vi "NI VeriStand - Timing Engine Globals.vi"() -> ()   [LabVIEW 2010, in "NI_VS FPGA Clock Support.lvlib"]
uses:
  <userlib>/_NI VeriStand FPGA Support/NI VeriStand FPGA Clock Support/NI_VS FPGA Clock Support.lvlib
panel:
  in  "Clock Pulse":bool
  in  "Clock Ticked":bool
  # "Internal Controls"
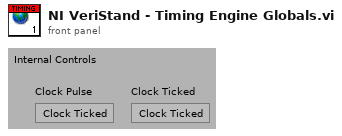
[diagram p1: front panel]
diagram:
